vi "FA_WriteETag.vi"(6 "Error In":errorcluster, 7 "eTag Value":string, 8 "ID":string) -> (0 "Error Out":errorcluster)   [LabVIEW 2014, in "FA_LocalStore.lvlib"]
doc: "Given a Special Type this VI writes a new eTag for that special type to the LocalStore."
uses:
  FA_LocalStore.lvlib
  <vilib>/Utility/config.llb/Write Key (String).vi
  <vilib>/Utility/config.llb/NI_LVConfig.lvlib
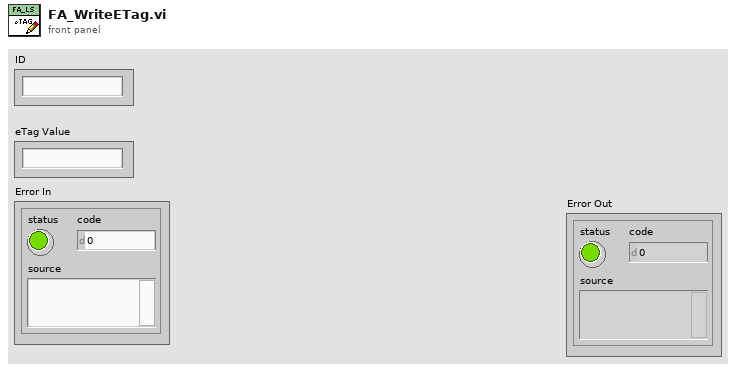
[diagram p1: front panel]
types:
  T1 = typedef "FA_LocalStore.lvlib/FA_LSRef.ctl" = cluster{"eTag INI Refnum":T2, "XML Refnum Array":refnum<file>[]}
  T2 = typedef "NI_LVConfig.lvlib/Config Data RefNum.ctl" = refnum<k1>
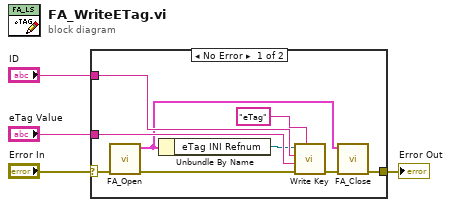
[diagram p0: block diagram]
diagram:
  n1 = case shown="No Error" "Error In" {
    selector: "Error In" -> [w7 w14]
    tunnel: [w9 w14] -> w4
    tunnel: "ID" -> [w11 _]
    tunnel: "eTag Value" -> [w12 _]
    frame No Error {
      n2 = call "FA_Open.vi"("Error In"=w7) -> ("Error Out"=w6:errorcluster, "FA_LS Ref"=w5:T1)  [unwired: 9 in]
      n3 = Unbundle By Name(w5) -> ("eTag INI Refnum"=w8:T2)
      n4 = call-poly <vilib>:"Write Key.vi"("section"="eTag", "error in (no error)"=w6, "value"=w12, "key"=w11, "refnum"=w8) -> ("error out"=w10:errorcluster)  [unwired: 4 in, 2 out]
      n5 = call "FA_Close.vi"("Error In"=w10, "FA_LS Ref"=w5) -> ("Error Out"=w9:errorcluster)  [unwired: 9 in]
    }
    frame Error {
    }
  }
  "Error Out" <- w4
